vi "FFT Co-processor (Host).vi"() -> ()   [LabVIEW 2014]
doc: "Uses the FPGA target as a co-processor that continuously computes the FFT of the user controlled signal.\n\nThe three signal are generated, added together, and sent through a DMA FIFO to the FPGA target. The data is then placed in a target-scoped FIFO and sent to the FFT Express VI, where the FFT of the data is computed. The FFT signal is then placed in a target-scoped FIFO and written back to the host through a DMA FIFO. The resulting FFT data is scaled and displayed on the host front panel."
uses:
  <vilib>/rvi/interface/RandomDataEmulation/nirviRandomDataOpen.vi
  <vilib>/rvi/interface/RandomDataEmulation/nirviRandomDataDMAMethods.vi
  <vilib>/rvi/interface/RandomDataEmulation/nirviRandomDataClose.vi
  <vilib>/rvi/interface/nirviOpenFPGA/nirviOpenFPGA.xnode
  FFT Co-processor (FPGA).vi
  <vilib>/rvi/interface/nirviMethod/nirviMethod.xnode
  <vilib>/rvi/interface/nirviCloseFPGA/nirviCloseFPGA.xnode
panel:
  out "Error":csg[](array[numeric])
  out "FFT Out":csg[](array[numeric])
  out "Receiving Loop":i32
  in  "Expected FFT {X}":csg[](array[numeric]) format="%.7g"
  out "Im min value":sgl=-0.007901356 format="%_15g"
  out "Im max value":sgl=0.007893026 format="%_15g"
  out "Re min value":sgl=-0.007883521 format="%_15g"
  out "Re max value":sgl=0.007913893 format="%_15g"
  in  "Chirped Data":csg[](array[numeric])
  in  "Knob":dbl(knob) scale=0.0..10.0
  in  "Send":bool
  out "Difference":i32
  out "data in":i32
  out "data out":i32
  # "16384"
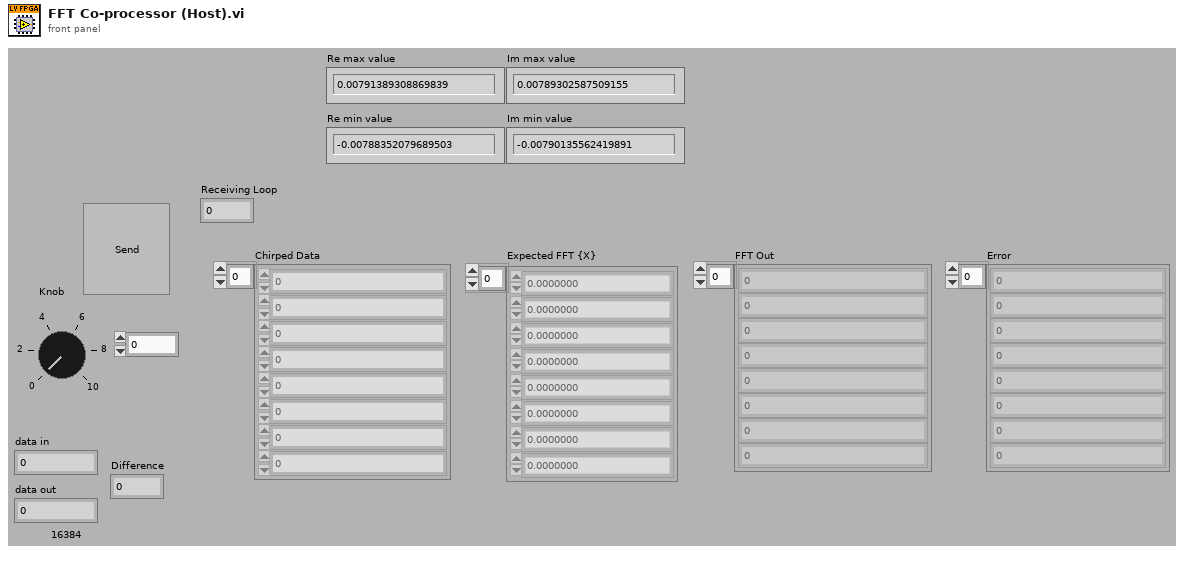
[diagram p1: front panel]
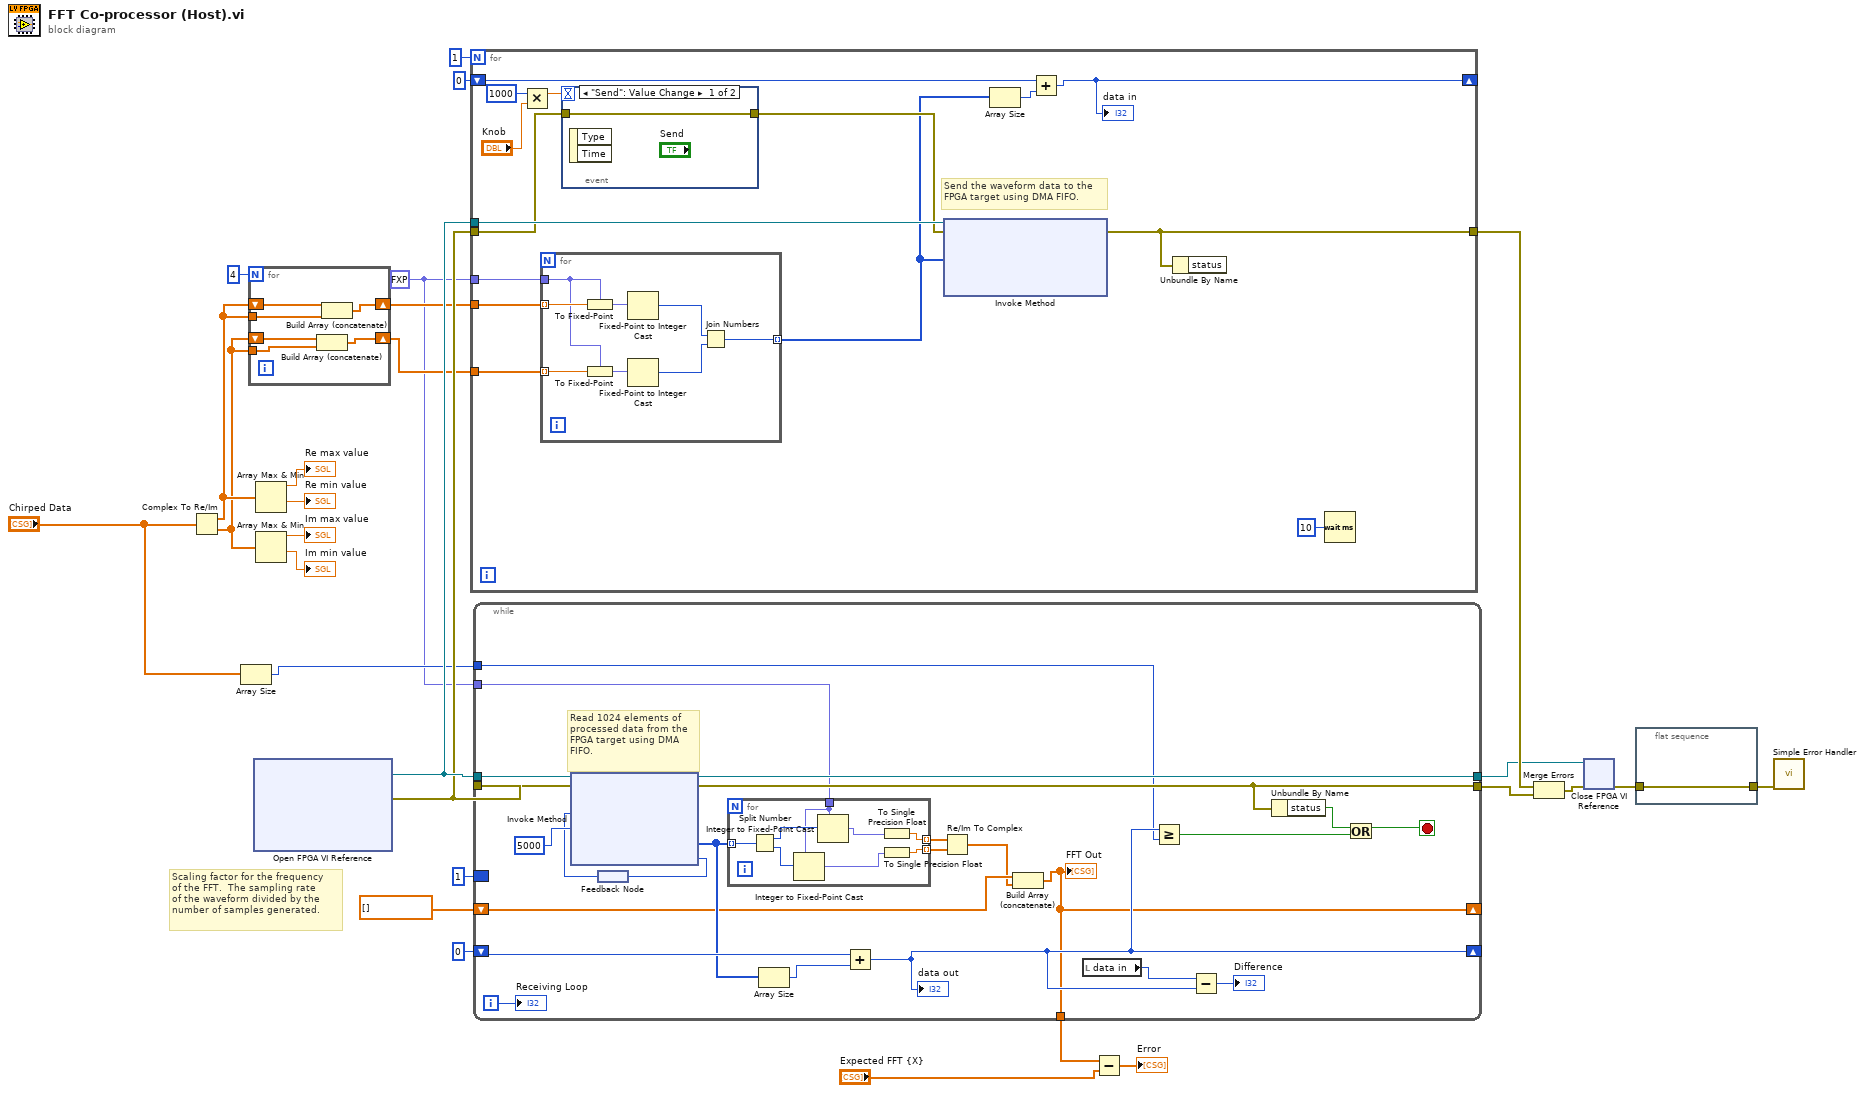
[diagram p0: block diagram]
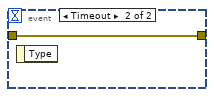
[diagram p2: hidden frame]
diagram:
  w4 = fxp<+/-,24,0> 0.0 ("real data in")
  # "Scaling factor for the frequency \nof the FFT.  The sampling rate \nof the waveform divided by the \nnumber of samples generated."
  n1 = Complex To Re/Im(x + iy="Chirped Data") -> (x=w13:sgl[], y=w12:sgl[])
  n2 = Array Size(array="Chirped Data") -> (size(s)=w5:i32)
  n3 = for {
    N: 4 -> [_]
    shift-right: [w30] -> w11
    shift-left: w13 -> [w34]
    shift-right: [w29] -> w10
    shift-left: w12 -> [w32]
    tunnel: w13 -> [w33]
    tunnel: w12 -> [w31]
    n4 = Build Array (concatenate)(w32, w31) -> (w29:sgl[])
    n5 = Build Array (concatenate)(w34, w33) -> (w30:sgl[])
  }
  n6 = xnode "Open FPGA VI Reference"() -> ("FPGA VI Reference Out"=w28:refnum<k20>, "error out"=w27:errorcluster)  [unwired: 2 in]
  n7 = Array Max & Min(array=w13) -> (max value=→"Re max value":sgl, min value=→"Re min value":sgl)  [unwired: 2 out]
  n8 = Array Max & Min(array=w12) -> (max value=→"Im max value":sgl, min value=→"Im min value":sgl)  [unwired: 2 out]
  n9 = for {
    N: 1 -> [_]
    tunnel: w28 -> [w49]
    tunnel: w27 -> [w44]
    tunnel: [w48] -> w25
    shift-right: [w45] -> _
    shift-left: 0 -> [w46]
    tunnel: w11 -> [w38]
    tunnel: w10 -> [w37]
    tunnel: w4 -> [w35]
    # "Send the waveform data to the\nFPGA target using DMA FIFO."
    n10 = Multiply(x=1000, y="Knob") -> (x*y=w41:dbl)
    n11 = for {
      tunnel: w38 -> [w57] mode=indexing
      tunnel: w37 -> [w53] mode=indexing
      tunnel: [w51] -> w36 mode=indexing
      tunnel: w35 -> [w50]
      n12 = To Fixed-Point(fixed-point type=w50, number=w57) -> (fixed-point=w56:fxp<+/-,24,0>)
      n13 = To Fixed-Point(fixed-point type=w50, number=w53) -> (fixed-point=w54:fxp<+/-,24,0>)
      n14 = Fixed-Point to Integer Cast(1:w56) -> (0:w55:i32)
      n15 = Fixed-Point to Integer Cast(1:w54) -> (0:w52:i32)
      n16 = Join Numbers(hi=w55, lo=w52) -> ((hi.lo)=w51:u64)
    }
    n17 = event shown="[0] \"Send\": Value Change" {
      selector: _ -> [_ _]
      dyn-events: _ -> [_ _]
      timeout: w41 -> [_ _]
      tunnel: w44 -> [w58 w59]
      tunnel: [w58 w59] -> w43
      event "Send": Value Change {
        n18 = event-data() -> ()  [unwired: 1 in, 2 out]
      }
      event Timeout {
        n19 = event-data() -> ()  [unwired: 1 in, 1 out]
      }
    }
    n20 = xnode "Invoke Method"("FPGA VI Reference In"=w49, "error in"=w43, "Data"=w36) -> ("error out"=w48:errorcluster)  [unwired: 1 in, 2 out]
    n21 = Array Size(array=w36) -> (size(s)=w47:i32)
    n22 = Add(x=w46, y=w47) -> (x+y=w45:i32)
    "data in" <- w45
    n23 = Unbundle By Name(w48) -> ()  [unwired: 1 out]
    n24 = Wait (ms)(milliseconds to wait=u32 10) -> ()  [unwired: 1 out]
  }
  n25 = while {
    tunnel: w28 -> [w82]
    tunnel: w27 -> [w81]
    tunnel: [w83] -> w23
    tunnel: [w79] -> w26
    shift-right: [w64] -> _
    shift-left: 0 -> [w78]
    border: u32 1 ("Elements Remaining") -> [_]
    shift-right: [w60] -> _
    shift-left: csg[] [] ("FFT Out") -> [w67]
    tunnel: w5 -> [w62]
    tunnel: w4 -> [w61]
    tunnel: [w60] -> w3
    i -> [w68]
    stop <- w80 stop-if-true
    # "Read 1024 elements of\nprocessed data from the\nFPGA target using DMA\nFIFO."
    n26 = feedback #1() -> (w69:u32)
    n27 = xnode "Invoke Method"("FPGA VI Reference In"=w82, "error in"=w81, "Number of Elements"=w69, "Timeout (ms)"=5000) -> ("FPGA VI Reference Out"=w83:refnum<k20>, "error out"=w79:errorcluster, "Data"=w77:u64[], "Elements Remaining"=w70:u32)
    n28 = feedback-in #1(w70) -> ()
    n29 = for {
      tunnel: w77 -> [w91] mode=indexing
      tunnel: [w90] -> w72 mode=indexing
      tunnel: [w89] -> w71 mode=indexing
      tunnel: w61 -> [w86]
      n30 = Split Number(x=w91) -> (hi(x)=w88:u32, lo(x)=w87:u32)
      n31 = Integer to Fixed-Point Cast(fixed-point type=w86, integer=w87) -> (fixed-point=w84:fxp<+/-,24,0>)
      n32 = Integer to Fixed-Point Cast(fixed-point type=w86, integer=w88) -> (fixed-point=w85:fxp<+/-,24,0>)
      n33 = To Single Precision Float(number=w85) -> (single precision float=w90:sgl)
      n34 = To Single Precision Float(number=w84) -> (single precision float=w89:sgl)
    }
    n35 = Array Size(array=w77) -> (size(s)=w76:i32)
    n36 = Add(x=w78, y=w76) -> (x+y=w64:i32)
    "data out" <- w64
    n37 = Re/Im To Complex(1:w71, 2:w72) -> (0:w66:csg[])
    n38 = Build Array (concatenate)(w67, w66) -> (w60:csg[])
    "FFT Out" <- w60
    n39 = local read "data in"() -> (w75:i32)
    n40 = Greater Or Equal?(x=w64, y=w62) -> (x >= y?=w65:bool)
    n41 = Subtract(x=w75, y=w64) -> (x-y=→"Difference":i32)
    n42 = Unbundle By Name(w79) -> ("status"=w63:bool)
    n43 = Or(x=w63, y=w65) -> (x .or. y?=w80:bool)
    "Receiving Loop" <- w68
  }
  n44 = Subtract(x=w3, y="Expected FFT {X}") -> (x-y=→"Error":csg[])
  n45 = Merge Errors(w25, w26) -> (w24:errorcluster)
  n46 = xnode "Close FPGA VI Reference"("FPGA VI Reference In"=w23, "error in"=w24) -> ("error out"=w22:errorcluster)
  n47 = flat-sequence {
    tunnel: w22 -> [w92]
    tunnel: [w92] -> w21
    frame #0 {
    }
  }
  n48 = call <vilib>:"Simple Error Handler.vi"("error in (no error)"=w21) -> ()  [unwired: 1 in, 8 out]
